vi "Read flow control.vi"(8 "error in (no error)":errorcluster, 11 "Serial Data Unit in":refnum<class "Serial Data Unit.lvclass">) -> (0 "error out":errorcluster, 2 "flow control":T1(ring), 3 "Serial Data Unit out":refnum<class "Serial Data Unit.lvclass">)   [LabVIEW 2021, in "Serial Data Unit.lvclass"]
uses:
  Serial Data Unit.lvclass
  Serial Data Unit.lvclass/Serial Data Unit.ctl
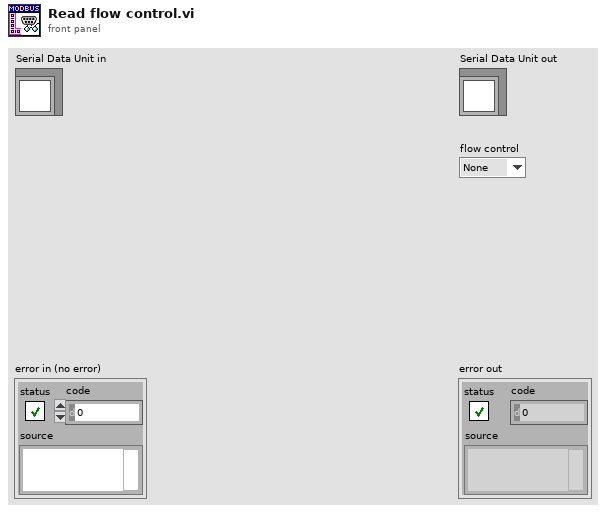
[diagram p1: front panel]
types:
  T1 = enum16{"None", "XON/XOFF", "RTS/CTS", "XON/XOFF & RTS/CTS", "DTR/DSR", "XON/XOFF & DTR/DSR"}
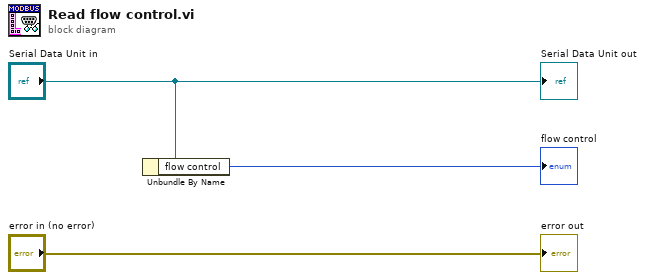
[diagram p0: block diagram]
diagram:
  n1 = Unbundle By Name("Serial Data Unit in") -> ("flow control"=→"flow control":T1)
  "error out" <- "error in (no error)"
  "Serial Data Unit out" <- "Serial Data Unit in"
